vi "status.vi"(8 "error in (no error)":errorcluster, 11 "EventDaemon in":refnum<class "TemplateDaemon.lvclass">) -> (0 "error out":errorcluster, 2 "status":T1, 3 "EventDaemon out":refnum<class "TemplateDaemon.lvclass">)   [LabVIEW 2024, in "TemplateDaemon.lvclass"]
doc: "Get current status and send via notifier."
uses:
  TemplateDaemon.lvclass
  status--cluster.ctl
  states--enum.ctl
  TemplateDaemon.lvclass/TemplateDaemon.ctl
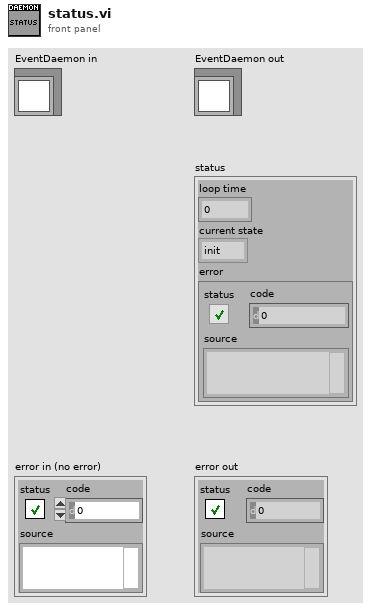
[diagram p1: front panel]
types:
  T1 = typedef "TemplateDaemon.lvclass/status--cluster.ctl" = cluster{"loop time":u32, "current state":T2, "error":errorcluster}
  T2 = typedef "TemplateDaemon.lvclass/states--enum.ctl" = enum16{"init", "default", "error handler", "exit"}
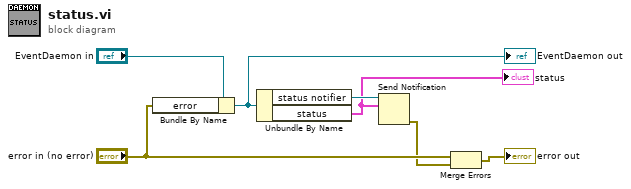
[diagram p0: block diagram]
diagram:
  n1 = Bundle By Name(cluster="EventDaemon in", "error"="error in (no error)") -> (w4:refnum<class "TemplateDaemon.lvclass">)
  "EventDaemon out" <- w4
  n2 = Unbundle By Name(w4) -> ("status notifier"=w7:refnum<notifier>, "status"=w6:T1)
  "status" <- w6
  n3 = Send Notification(notification=w6, notifier=w7) -> (error out=w1:errorcluster)  [unwired: 1 in, 1 out]
  n4 = Merge Errors("error in (no error)", w1) -> (→"error out":errorcluster)
